vi "DataStream_RetrieveA.vi"(4 "BytesToCombine (4)":i32=4, 5 "error in (no error)":errorcluster, 6 "data file pointer":u32, 7 "transferSize":i32, 8 "no. of channels":i32) -> (0 "error out":errorcluster, 1 "Rcvd Pts/CH":i32, 2 "Debug Data":cluster{"4byte word":u8[], "word":u32}[](array[cluster]), 3 "32bit data":u32[](array[numeric]))   [LabVIEW 2010, in "lib1299.lvlib"]
doc: "This VI reads the requested number of points from the data file provided and combines the 8-bit values to a 32-bit word.\n\nInputs:\nNo of channels - number of channels\ntransferSize - number of points to read from the data file\ndata file pointer - pointer to the data file\nBytesToCombine - number of bytes to combine into a word (default = 4)\nerror in - error input cluster\n\nOutputs:\nError out - error output cluster\n32bits data - array of data in 32bit format\nDebugData - cluster output for writing to debug file\n - 4byte word: 4 bytes (word) read, hex format\n - word - combined 4 bytes in decimal"
uses:
  lib1299.lvlib
panel:
  out "Pts rcvd":i32
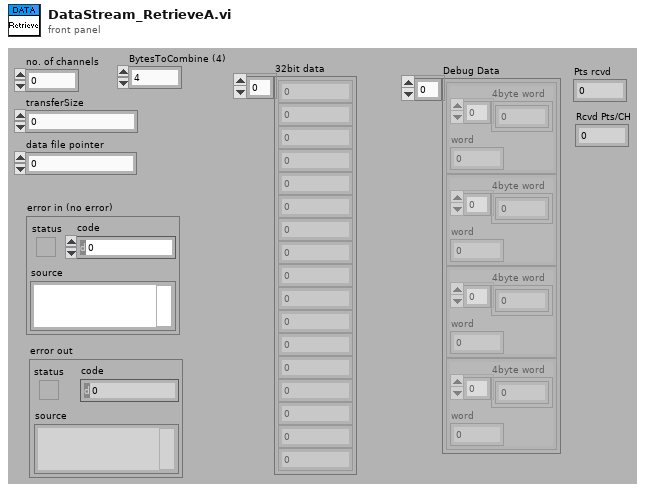
[diagram p1: front panel]
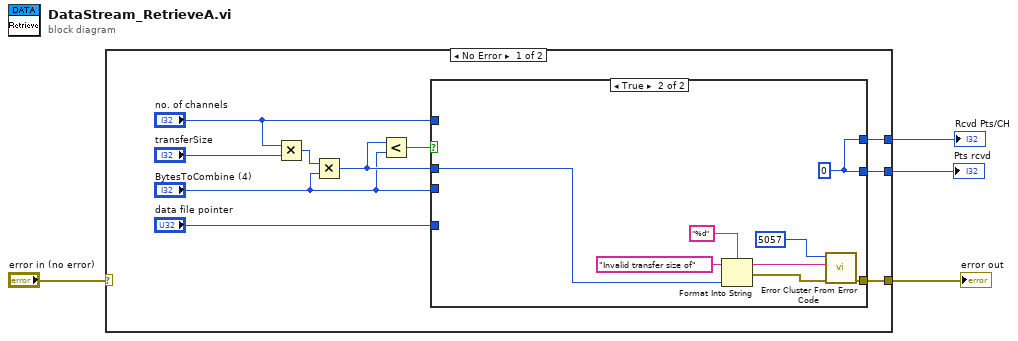
[diagram p0: block diagram]
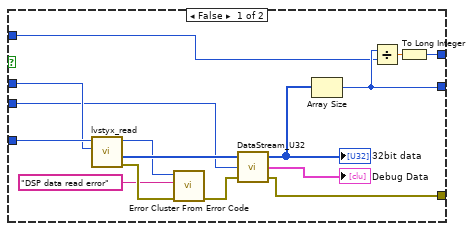
[diagram p2: hidden frame]
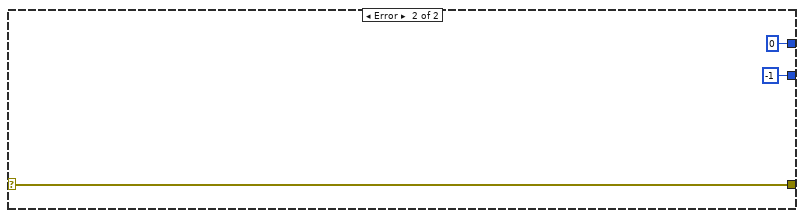
[diagram p3: hidden frame]
diagram:
  n1 = case shown="No Error" "error in (no error)" {
    selector: "error in (no error)" -> [_ w40]
    tunnel: [w11 w40] -> w3
    tunnel: [w7 -1] -> w2
    tunnel: [w5 0] -> w1
    frame No Error {
      n2 = Multiply(x="no. of channels", y="transferSize") -> (x*y=w12:i32)
      n3 = Multiply(x=w12, y="BytesToCombine (4)") -> (x*y=w10:i32)
      n4 = Less?(x=w10, y="BytesToCombine (4)") -> (x < y?=w8:bool)
      n5 = case shown="True" w8 {
        tunnel: "data file pointer" -> [w28 _]
        tunnel: [w27 w37] -> w11
        tunnel: w10 -> [w21 w32]
        tunnel: "BytesToCombine (4)" -> [w20 _]
        tunnel: [w18 w30] -> w7
        tunnel: "no. of channels" -> [w17 _]
        tunnel: [w15 w30] -> w5
        frame False {
          n6 = call "lvstyx_read.vi"("requested length"=w21, "file ptr"=w28) -> ("error out"=w25:errorcluster, "data"=w26:i8[], "result"=w23:i32)  [unwired: 6 in, 1 out]
          n7 = call <vilib>:"Error Cluster From Error Code.vi"("error in (no error)"=w25, "error message (\"\")"="DSP data read error" ("error message (\"\")"), "error code (0)"=w23) -> ("error out"=w24:errorcluster)  [unwired: 6 in]
          n8 = call "DataStream_U32.vi"("error in (no error)"=w24, "BytesToCombine"=w20, "data buffer"=w26) -> ("error out"=w27:errorcluster, "Debug Data"=→"Debug Data":cluster{"4byte word":u8[], "word":u32}[], "32bit data"=w19:u32[])
          "32bit data" <- w19
          n9 = Array Size(array=w19) -> (size(s)=w18:i32)
          n10 = Divide(x=w18, y=w17) -> (x/y=w16:dbl)
          n11 = To Long Integer(number=w16) -> (32bit integer=w15:i32)
        }
        frame True {
          w30 = 0
          n12 = Format Into String(format string="%d", initial string="Invalid transfer size of", w32) -> (resulting string=w35:string, error out=w31:errorcluster)  [unwired: 1 in]
          n13 = call <vilib>:"Error Cluster From Error Code.vi"("error in (no error)"=w31, "error message (\"\")"=w35, "error code (0)"=5057) -> ("error out"=w37:errorcluster)  [unwired: 6 in]
        }
      }
    }
    frame Error {
    }
  }
  "error out" <- w3
  "Pts rcvd" <- w2
  "Rcvd Pts/CH" <- w1
